vi "Jednoręki Bandyta.vi"() -> ()   [LabVIEW 2020]
panel:
  out "Wynik!":string
  out "3":dbl
  in  "stop 3":bool
  out "2":dbl
  in  "stop 2":bool
  out "1":dbl
  in  "stop":bool
  in  "Start":bool
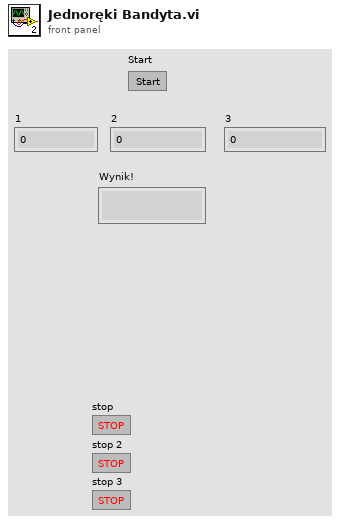
[diagram p1: front panel]
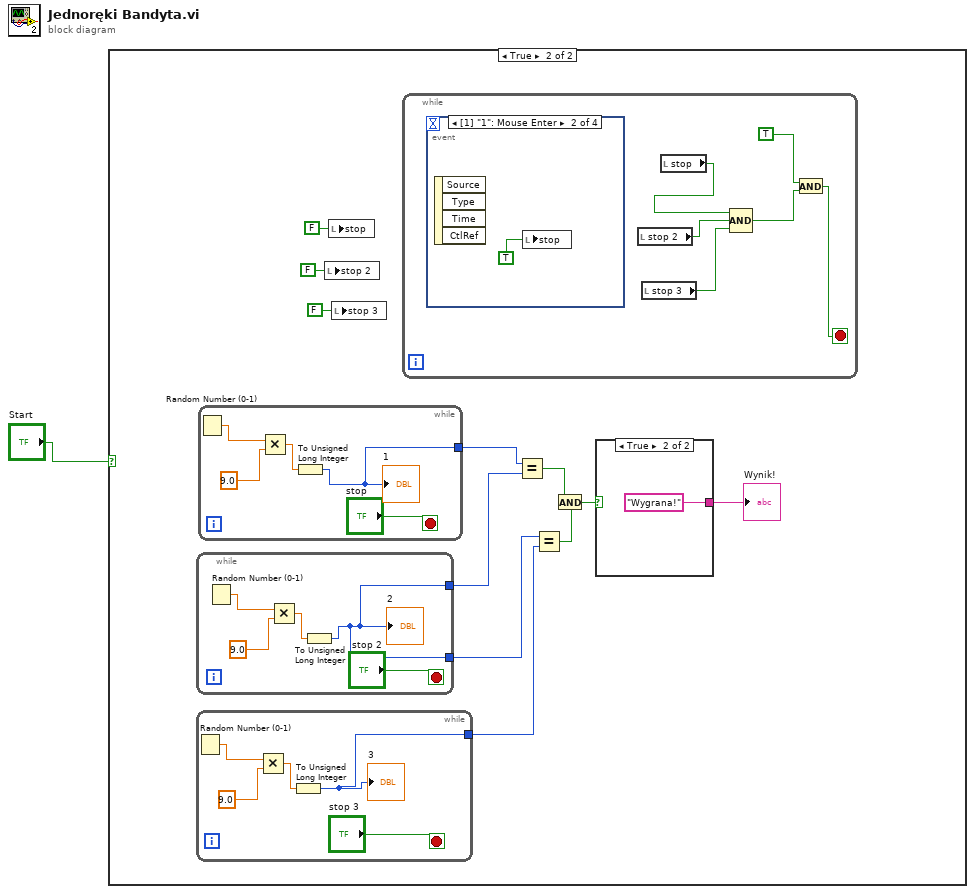
[diagram p0: block diagram]
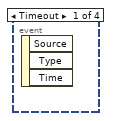
[diagram p3: hidden frame]
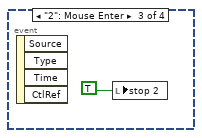
[diagram p4: hidden frame]
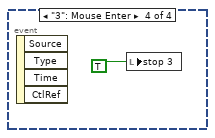
[diagram p5: hidden frame]
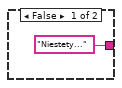
[diagram p6: hidden frame]
diagram:
  n1 = case shown="True" "Start" {
    frame False {
    }
    frame True {
      n2 = while {
        tunnel: [w30] -> w11
        tunnel: [w30] -> w10
        stop <- "stop 2" stop-if-true
        n3 = Random Number (0-1)() -> (number: 0 to 1=w33:dbl)
        n4 = Multiply(x=w33, y=9.0) -> (x*y=w32:dbl)
        n5 = To Unsigned Long Integer(number=w32) -> (unsigned 32bit integer=w30:u32)
        "2" <- w30
      }
      n6 = while {
        tunnel: [w25] -> w9
        stop <- "stop 3" stop-if-true
        n7 = Random Number (0-1)() -> (number: 0 to 1=w27:dbl)
        n8 = Multiply(x=w27, y=9.0) -> (x*y=w28:dbl)
        n9 = To Unsigned Long Integer(number=w28) -> (unsigned 32bit integer=w25:u32)
        "3" <- w25
      }
      n10 = while {
        tunnel: [w35] -> w12
        stop <- "stop" stop-if-true
        n11 = Random Number (0-1)() -> (number: 0 to 1=w37:dbl)
        n12 = Multiply(x=w37, y=9.0) -> (x*y=w38:dbl)
        n13 = To Unsigned Long Integer(number=w38) -> (unsigned 32bit integer=w35:u32)
        "1" <- w35
      }
      n14 = local write "stop 2"(FALSE ("stop 2")) -> ()
      n15 = local write "stop"(FALSE ("stop")) -> ()
      n16 = local write "stop 3"(FALSE ("stop 3")) -> ()
      n17 = while {
        stop <- w15 stop-if-true
        n18 = event shown="[1] \"1\": Mouse Enter" {
          selector: _ -> [_ _ _ _]
          dyn-events: _ -> [_ _ _ _]
          timeout: _ -> [_ _ _ _]
          event Timeout {
            n19 = event-data() -> ()  [unwired: 1 in, 3 out]
          }
          event "1": Mouse Enter {
            n20 = event-data() -> ()  [unwired: 1 in, 4 out]
            n21 = local write "stop"(TRUE ("stop")) -> ()
          }
          event "2": Mouse Enter {
            n22 = event-data() -> ()  [unwired: 1 in, 4 out]
            n23 = local write "stop 2"(TRUE ("stop 2")) -> ()
          }
          event "3": Mouse Enter {
            n24 = event-data() -> ()  [unwired: 1 in, 4 out]
            n25 = local write "stop 3"(TRUE ("stop 3")) -> ()
          }
        }
        n26 = local read "stop 2"() -> (w16:bool)
        n27 = local read "stop 3"() -> (w17:bool)
        n28 = local read "stop"() -> (w18:bool)
        n29 = Compound Arithmetic op=AND(w18, w16, w17) -> (w13:bool)
        n30 = And(x=TRUE, y=w13) -> (x .and. y?=w15:bool)
      }
      n31 = Equal?(x=w12, y=w11) -> (x = y?=w7:bool)
      n32 = Equal?(x=w10, y=w9) -> (x = y?=w6:bool)
      n33 = And(x=w7, y=w6) -> (x .and. y?=w8:bool)
      n34 = case shown="True" w8 {
        tunnel: ["Niestety..." ("String") "Wygrana!"] -> w5
        frame False {
        }
        frame True {
        }
      }
      "Wynik!" <- w5
    }
  }
